vi "Simplest.vi"() -> ()   [LabVIEW 2012]
doc: "Application example"
panel:
  out "LV ERROR OUT":errorcluster
  out "RESISTANCE":sgl format="%^_6e"
  out "DVM OVR":bool=TRUE
  # "Simplest.vi"
  # "This VI is perhaps the easiest way to get a reading from the AVS-47B. \n\nOpen also the \"Manage Configuration File.vi\" and change its front panel controls\naccording to your needs. Verify that the VISA resource is correct: If you use a USB-232\nconverter, check with  NI MAX the name of the serial port that the converter imitates. \nSave the \"Create.....vi\" so that you need not change so many settings the next time.\n\nRun the \"Simplest.vi\". It should return the measured resistance value in ohms. This VI\ncan be run both in local and remote modes. It does not program the temperature\ncontroller and it interprets all readings as resistances regardless of the  position \nof the DISPLAY switch. \n\nThis simple application example VI was not designed for being run continuously. \nEvery time it is run, it opens the VISA session and closes it when exiting."
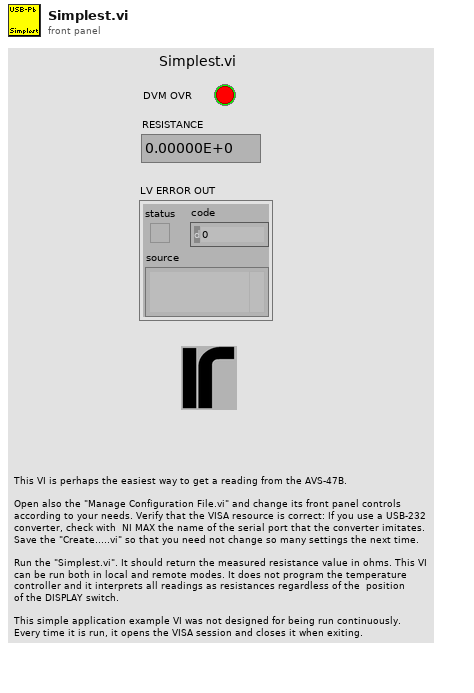
[diagram p1: front panel]
types:
  T1 = cluster{"VISA RESOURCE":refnum<visa-resource-name>, "PICOBUS ADDRESS":u8, "DISABLE AL":u8, "REMOTE":u8, "INPUT":u8, "CHANNEL":u8, "RANGE":u8, "EXCITATION":u8, "DISPLAY":u8, "DIGITAL REFERENCE":u16, "SET POINT":dbl, "PROP GAIN":u8, "INTG":u8, "DERIV":u8, "POWER BIAS":u8, "POWER RANGE":u8, "INFO STRING":string, "HEATER RESISTANCE":dbl, "INTERVAL":u8, " SENSOR dR/dT":u8}
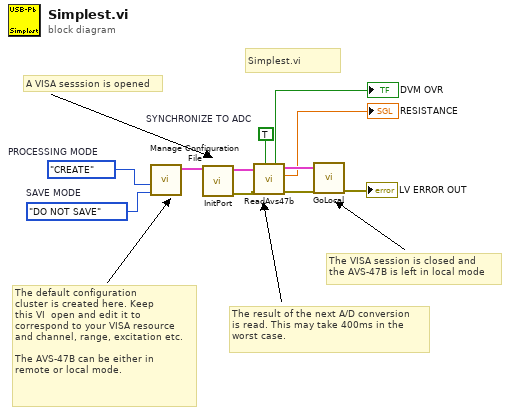
[diagram p0: block diagram]
diagram:
  w1 = enum16{"DO NOT SAVE", "SAVE .CNF FILE"}."DO NOT SAVE"  # SAVE MODE
  w2 = enum16{"NONE", "READ", "CREATE"}."CREATE"  # PROCESSING MODE
  w9 = TRUE  # SYNCHRONIZE TO ADC
  # "A VISA sesssion is opened"
  # "The VISA session is closed and\nthe AVS-47B is left in local mode"
  # "The result of the next A/D conversion\nis read. This may take 400ms in the\nworst case."
  # "The default configuration\ncluster is created here. Keep\nthis VI  open and edit it to \ncorrespond to your VISA resource \nand channel, range, excitation etc.\n\nThe AVS-47B can be either in\nremote or local mode."
  # "Simplest.vi"
  n1 = call "Manage Configuration File.vi"("SAVE MODE"=w1, "PROCESSING MODE"=w2) -> ("CONFIGURATION CLUSTER OUT"=w5:T1)  [unwired: 9 in]
  n2 = call "InitPort.vi"("CONFIGURATION CLUSTER"=w5) -> ("LV ERROR OUT"=w3:errorcluster, "UNMODIFIED CONFIGURATION CLUSTER"=w4:T1)  [unwired: 6 in, 1 out]
  n3 = call "ReadAvs47b.vi"("SYNCHRONISE TO ADC"=w9, "LV ERROR IN"=w3, "CONFIGURATION CLUSTER"=w4) -> ("LV ERROR OUT"=w10:errorcluster, "RESISTANCE (OHMS)"=→"RESISTANCE":sgl, "MODIFIED CONFIGURATION CLUSTER"=w11:T1, "ADC OVERRANGE"=→"DVM OVR":bool)  [unwired: 3 in, 2 out]
  n4 = call "GoLocal.vi"("LV ERROR IN"=w10, "CONFIGURATION CLUSTER"=w11) -> ("LV ERROR OUT"=→"LV ERROR OUT":errorcluster)  [unwired: 9 in]
